vi "Hex2String.vi"(1 "Hex":string) -> (0 "String":string)   [LabVIEW 2012]
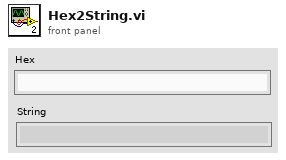
[diagram p1: front panel]
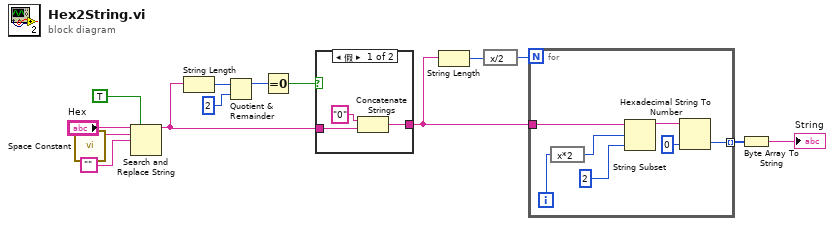
[diagram p0: block diagram]
diagram:
  n1 = call <vilib>:"Space Constant.vi"() -> ("String"=w2:string)
  n2 = Search and Replace String(replace all?=TRUE ("替换全部？(F)"), input string="Hex", search string=w2, replace string="") -> (result string=w4:string)  [unwired: 4 in, 3 out]
  n3 = String Length(string=w4) -> (length=w14:i32)
  n4 = Quotient & Remainder(x=w14, y=2) -> (x-y*floor(x/y)=w12:i32)  [unwired: 1 out]
  n5 = Equal To 0?(x=w12) -> (x = 0?=w11:bool)
  n6 = case shown="假" w11 {
    tunnel: w4 -> [w17 w18]
    tunnel: [w15 w18] -> w10
    frame False {
      n7 = Concatenate Strings("0" ("字符串"), w17) -> (w15:string)
    }
    frame True {
    }
  }
  n8 = String Length(string=w10) -> (length=w9:i32)
  n9 = expression code="x/2"(w9) -> (w8:i32)
  n10 = for {
    N: w8 -> [_]
    tunnel: w10 -> [w25]
    tunnel: [w19] -> w7 mode=indexing
    i -> [w23]
    n11 = expression code="x*2"(w23) -> (w22:i32)
    n12 = String Subset(string=w25, offset (0)=w22, length (rest)=2 ("长度（剩余）")) -> (substring=w21:string)
    n13 = Hexadecimal String To Number(string=w21, default (0uL)=u8 0 ("默认(0 U32)")) -> (number=w19:u8)  [unwired: 1 in, 1 out]
  }
  n14 = Byte Array To String(unsigned byte array=w7) -> (string=→"String":string)
